vi "config.vi"(5 "Function":enum16{"write", "read"}(ring), 6 "Error In":errorcluster, 7 "Instrument":T10 items=["SIMULATE", "CF900", "DR200", "MNK", "PPMS1", "PPMS2", "THz1", "THz2", "MFP3D", "CYPHER"], 8 "Amplifiers":T8, 9 "DAQ Type":T9, 10 "AO Configuration":T1, 11 "AI Configuration":T4) -> (0 "Amplifiers":T8, 1 "DAQ Type":T9, 2 "AO Configuration 2":T1, 3 "AI Configuration 2":T4, 4 "Error Out":errorcluster)   [LabVIEW 2016]
uses:
  Instrument.Lockin/Typedefs/AI.config(UI)-array.ctl
  Instrument.Lockin/Typedefs/AI.config(UI)-cluster.ctl
  Instrument.Lockin/Typedefs/AI.coupling-enum.ctl
  Instrument.Lockin/Typedefs/446xAI-enum.ctl
  Instrument.Lockin/Typedefs/AO.config(UI)-array.ctl
  Instrument.Lockin/Typedefs/AO.config(UI)-cluster.ctl
  Instrument.Lockin/Typedefs/446xAO-enum.ctl
  Instrument.Lockin/Typedefs/AmplifierType-enum.ctl
  Instrument.Lockin/Typedefs/DAQType-enum.ctl
  Instrument.Lockin/Typedefs/INI-enum.ctl
  Instrument.Lockin/Instrument.Lockin.lvclass
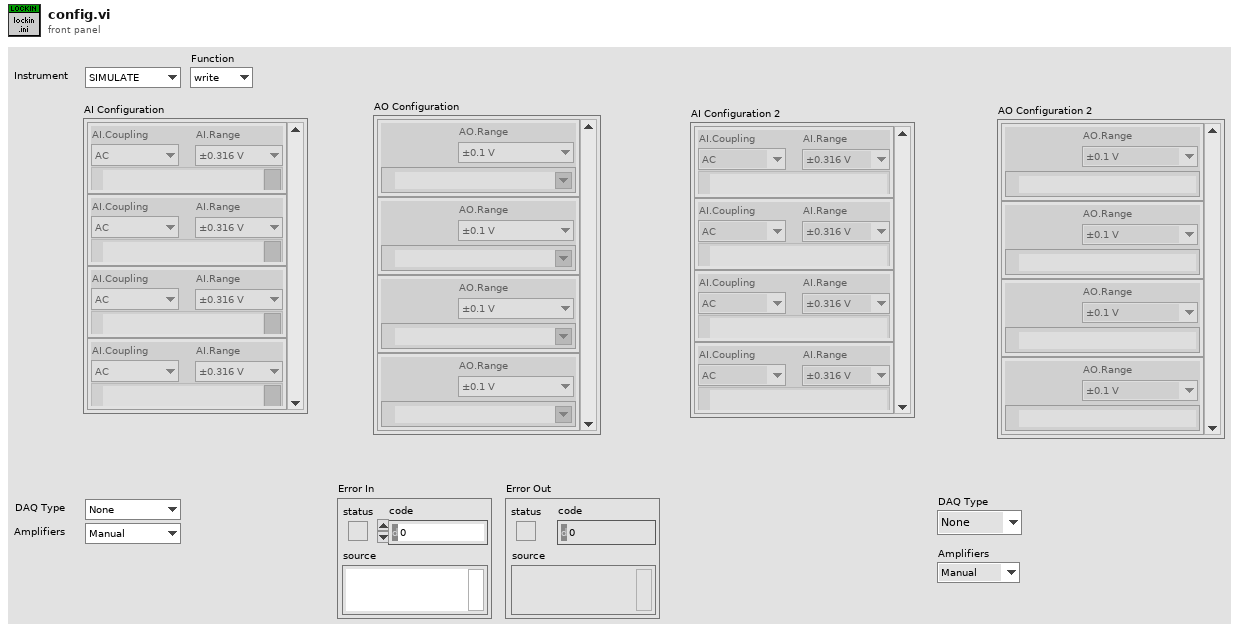
[diagram p1: front panel]
types:
  T1 = typedef "Instrument.Lockin.lvclass/AO.config(UI)-array.ctl" = T2[]
  T2 = typedef "Instrument.Lockin.lvclass/AO.config(UI)-cluster.ctl" = cluster{"AO.Range":T3, "AO.channels":tag}
  T3 = typedef "Instrument.Lockin.lvclass/446xAO-enum.ctl" = enum16{"±0.1 V", "±1.0 V", "±10.0 V"}
  T4 = typedef "Instrument.Lockin.lvclass/AI.config(UI)-array.ctl" = T5[]
  T5 = typedef "Instrument.Lockin.lvclass/AI.config(UI)-cluster.ctl" = cluster{"AI.Coupling":T6, "AI.channels":tag, "AI.Range":T7}
  T6 = typedef "Instrument.Lockin.lvclass/AI.coupling-enum.ctl" = enum16{"AC", "DC", "GND"}
  T7 = typedef "Instrument.Lockin.lvclass/446xAI-enum.ctl" = enum16{"±0.316 V", "±1.00 V", "±3.16 V", "±10.0 V", "±31.6 V", "±42.4 V"}
  T8 = typedef "Instrument.Lockin.lvclass/AmplifierType-enum.ctl" = enum16{"Manual", "Krohn Hite", "Femto"}
  T9 = typedef "Instrument.Lockin.lvclass/DAQType-enum.ctl" = enum16{"None", "USB 4431", "PXI 446x"}
  T10 = typedef "Instrument.Lockin.lvclass/INI-enum.ctl" = u16
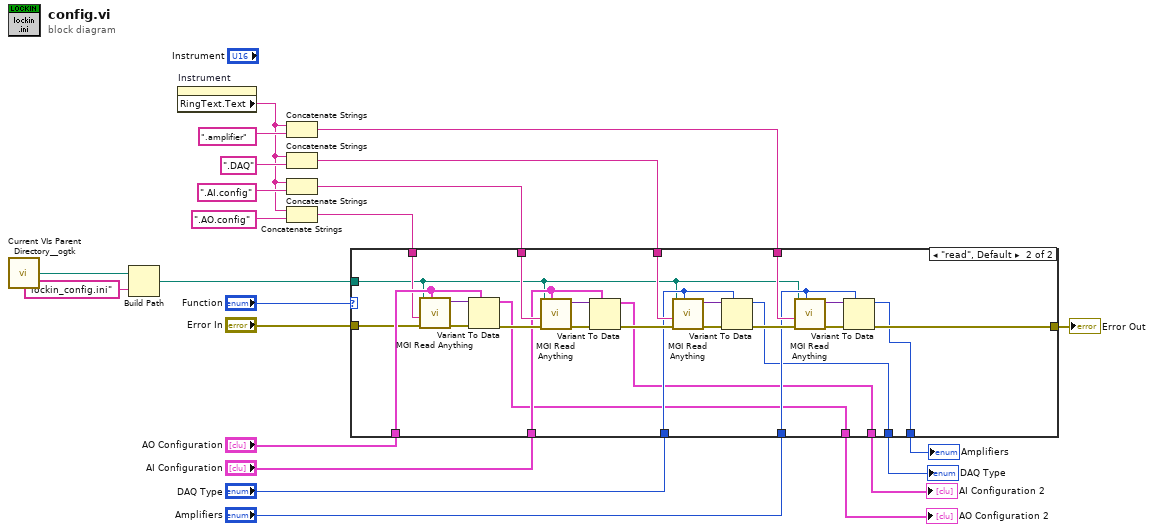
[diagram p0: block diagram]
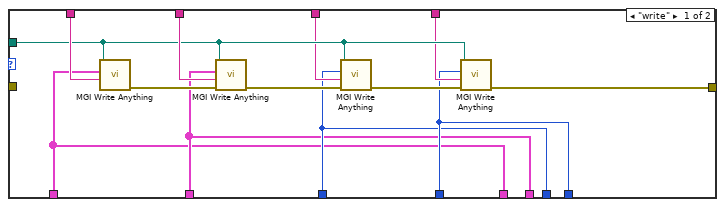
[diagram p2: hidden frame]
diagram:
  n1 = call <userlib>:"Current VIs Parent Directory__ogtk.vi"() -> ("Parent Directory (+ Relative)"=w1:path)  [unwired: 5 in]
  n2 = Build Path(base path=w1, name or relative path="lockin_config.ini") -> (appended path=w18:path)
  n3 = property on="Instrument" class="Ring (strict)"() -> ("RingText.Text"=w2:string)  [unwired: 2 in, 2 out]
  n4 = Concatenate Strings(w2, ".amplifier" ("Section Name (Name of \"Anything\")")) -> (w9:string)
  n5 = Concatenate Strings(w2, ".DAQ" ("Section Name (Name of \"Anything\")")) -> (w10:string)
  n6 = Concatenate Strings(w2, ".AI.config" ("Section Name (Name of \"Anything\")")) -> (w11:string)
  n7 = Concatenate Strings(w2, ".AO.config" ("Section Name (Name of \"Anything\")")) -> (w12:string)
  n8 = case shown="\"read\", Default" "Function" {
    tunnel: w12 -> [w36 w53]
    tunnel: "AI Configuration" -> [w25 w49]
    tunnel: w11 -> [w34 w52]
    tunnel: "AO Configuration" -> [w24 w60]
    tunnel: "DAQ Type" -> [w26 w48]
    tunnel: "Amplifiers" -> [w27 w46]
    tunnel: w18 -> [w31 w43]
    tunnel: [w30 w45] -> w17
    tunnel: w10 -> [w29 w51]
    tunnel: w9 -> [w28 w50]
    tunnel: "Error In" -> [_ w44]
    tunnel: [w24 w42] -> w6
    tunnel: [w25 w41] -> w5
    tunnel: [w26 w40] -> w4
    tunnel: [w27 w39] -> w3
    frame "write" {
      n9 = call <userlib>:"MGI Write Anything.vi"("Section Name (Name of \"Anything\")"=w36, "Anything"=w24, "Path (dialog)"=w31) -> ("Error Out"=w35:errorcluster)  [unwired: 6 in, 2 out]
      n10 = call <userlib>:"MGI Write Anything.vi"("Error In"=w35, "Section Name (Name of \"Anything\")"=w34, "Anything"=w25, "Path (dialog)"=w31) -> ("Error Out"=w33:errorcluster)  [unwired: 5 in, 2 out]
      n11 = call <userlib>:"MGI Write Anything.vi"("Error In"=w33, "Section Name (Name of \"Anything\")"=w29, "Anything"=w26, "Path (dialog)"=w31) -> ("Error Out"=w32:errorcluster)  [unwired: 5 in, 2 out]
      n12 = call <userlib>:"MGI Write Anything.vi"("Error In"=w32, "Section Name (Name of \"Anything\")"=w28, "Anything"=w27, "Path (dialog)"=w31) -> ("Error Out"=w30:errorcluster)  [unwired: 5 in, 2 out]
    }
    frame "read", Default {
      n13 = call <userlib>:"MGI Read Anything.vi"("Type of Anything"=w60, "Error In"=w44, "Section Name (Name of \"Type of Anything\")"=w53, "Path (dialog)"=w43) -> ("Error Out"=w62:errorcluster, "Anything"=w61:variant)  [unwired: 4 in, 2 out]
      n14 = Variant To Data(error in=w62, type=w60, Variant=w61) -> (data=w42:T1, error out=w58:errorcluster)
      n15 = call <userlib>:"MGI Read Anything.vi"("Type of Anything"=w49, "Error In"=w58, "Section Name (Name of \"Type of Anything\")"=w52, "Path (dialog)"=w43) -> ("Error Out"=w59:errorcluster, "Anything"=w37:variant)  [unwired: 4 in, 2 out]
      n16 = Variant To Data(error in=w59, type=w49, Variant=w37) -> (data=w41:T4, error out=w56:errorcluster)
      n17 = call <userlib>:"MGI Read Anything.vi"("Type of Anything"=w48, "Error In"=w56, "Section Name (Name of \"Type of Anything\")"=w51, "Path (dialog)"=w43) -> ("Error Out"=w57:errorcluster, "Anything"=w38:variant)  [unwired: 4 in, 2 out]
      n18 = Variant To Data(error in=w57, type=w48, Variant=w38) -> (data=w40:T9, error out=w54:errorcluster)
      n19 = call <userlib>:"MGI Read Anything.vi"("Type of Anything"=w46, "Error In"=w54, "Section Name (Name of \"Type of Anything\")"=w50, "Path (dialog)"=w43) -> ("Error Out"=w55:errorcluster, "Anything"=w47:variant)  [unwired: 4 in, 2 out]
      n20 = Variant To Data(error in=w55, type=w46, Variant=w47) -> (data=w39:T8, error out=w45:errorcluster)
    }
  }
  "Error Out" <- w17
  "AO Configuration 2" <- w6
  "AI Configuration 2" <- w5
  "DAQ Type" <- w4
  "Amplifiers" <- w3
